vi "Compute Square-Gated Discrete Calibration Phasor & jw.vi"(6 "Gate Width (W)":dbl[unit], 8 "Laser Period (T)":dbl[unit], 9 "Calibration Lifetime (tau)":dbl[unit], 10 "# Gates (N)":dbl, 11 "Harmonic frequency (f)":dbl[unit]) -> (2 "Z_N[W](tau)/Z_N[W](0)":cdb, 3 "i 2 pi f (GHz)":cdb)   [LabVIEW 2019]
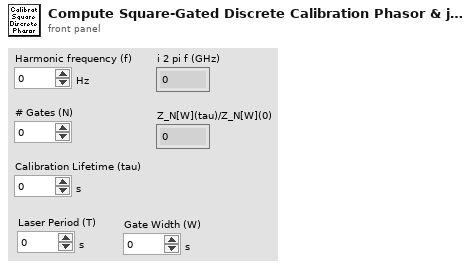
[diagram p1: front panel]
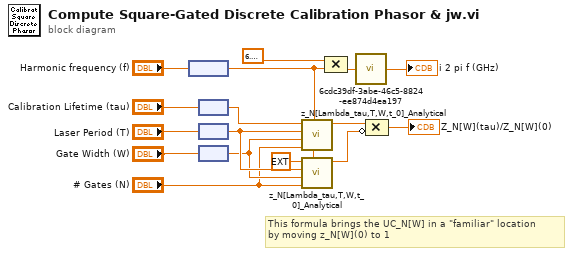
[diagram p0: block diagram]
diagram:
  # "This formula brings the UC_N[W] in a \"familiar\" location\nby moving z_N[W](0) to 1"
  n1 = node("Harmonic frequency (f)") -> (w1:dbl)
  n2 = node("Calibration Lifetime (tau)") -> (w8:dbl)
  n3 = node("Laser Period (T)") -> (w7:dbl)
  n4 = node("Gate Width (W)") -> (w6:dbl)
  n5 = call "z_N[Lambda_tau,T,W,t_0]_Analytical.vi"("Harmonic f"=w1, "N"="# Gates (N)", "W"=w6, "T"=w7, "tau"=w8) -> ("z_n,N,W(tau)"=w9:cxt)  [unwired: 6 in]
  n6 = call "z_N[Lambda_tau,T,W,t_0]_Analytical.vi"("Harmonic f"=w1, "N"="# Gates (N)", "W"=w6, "T"=w7, "tau"=ext 0.0) -> ("z_n,N,W(tau)"=w2:cxt)  [unwired: 6 in]
  n7 = Compound Arithmetic op=MULTIPLY(6.283185307179586, w1) -> (w16:dbl)
  n8 = call "6cdc39df-3abe-46c5-8824-ee874d4ea197.vi"("x (1)"=w16) -> ("ix"=→"i 2 pi f (GHz)":cdb)
  n9 = Compound Arithmetic op=MULTIPLY(w9, invert w2) -> (→"Z_N[W](tau)/Z_N[W](0)":cxt)
